vi "Configure Serial Bus (USBP - Trigger).vi"(0 "VISA resource name":refnum<visa-resource-name>, 1 "Control Message Type (0: Good CRC)":i32(ring) items=["Good CRC", "Goto Min", "Accept", "Reject", "Ping", "PS_RDY", "Get Source Cap", "Get Sink Cap", "DR Swap", "PR Swap", " VCONN Swap", "Wait", "Soft Reset", "Get Source Cap Extended ", "Get Status ", "FR Swap", "Get PPS Status ", "Get Country Codes "], 2 "Qualifier Type (0: None)":i32(ring) items=["None", "SOP", "SPR", "SDPR"], 5 "Serial Bus Name (1: Serial Bus 1)":i32(ring)=1 items=["Serial Bus 1"=1, "Serial Bus 2"=2], 7 "Trigger Mode (0: Preamble Start)":i32(ring) items=["Preamble Start", "End Of Packet", "SOP", "SP Rime", "SDP Rime", "SP Debug", "SDP Debug", "Hard Reset", "Cable Reset", "CRC Error", "Preamble Error", "Header Content"], 9 "Header Type (0: Control Message)":i32(ring) items=["Control Message", "Data Message", "Extended Message", " Value"], 11 "error in (no error)":errorcluster, 12 "Data Message Type (0: Source Capabilities)":i32(ring) items=["Source Capabilities", "Request", "BIST", "Sink Capabilities", "Battery Status", "Alert", "Get Country Info", "Vendor Defined"], 13 "Extended Message Type (0: Source Capabilities Extended )":i32(ring) items=["Source Capabilities Extended ", "Status", "Get Battery Cap", "Get Battery Status", "Battery Capabilities", "Get Manufacturer Info", "Manufacturer Info", "Security Request", "Security Response", "Firmware Update Request", "Firmware Update Response", "PPS Status", "Country Information", "Country Codes"], 14 "Header Value (XXXXXXXXXXXXXXXX)":string="XXXXXXXXXXXXXXXX") -> (4 "VISA resource name out":refnum<visa-resource-name>, 15 "error out":errorcluster)   [LabVIEW 2015, in "Agilent 2000 3000 X-Series.lvlib"]
doc: "Configures the trigger settings of USB Pd bus.\n\n<b>Note:</b>\nThis VI is only applicable for 3000T, 3000G, 4000 X-Series."
uses:
  Agilent 2000 3000 X-Series.lvlib
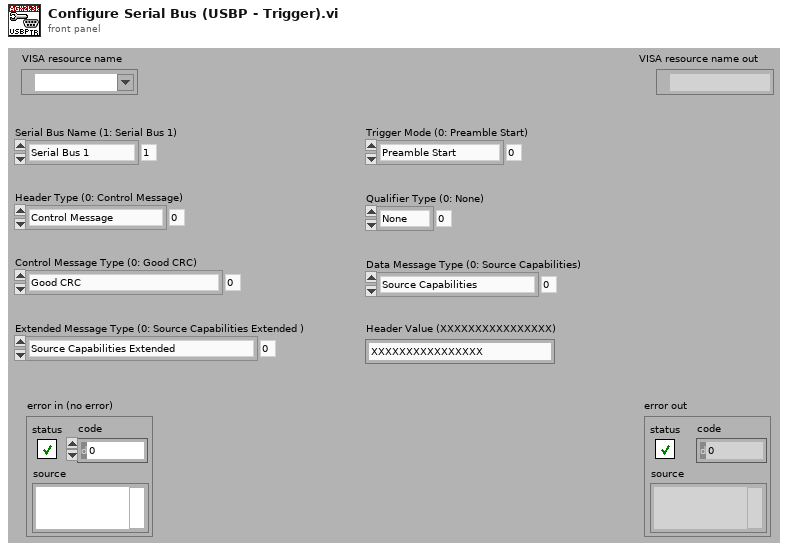
[diagram p1: front panel]
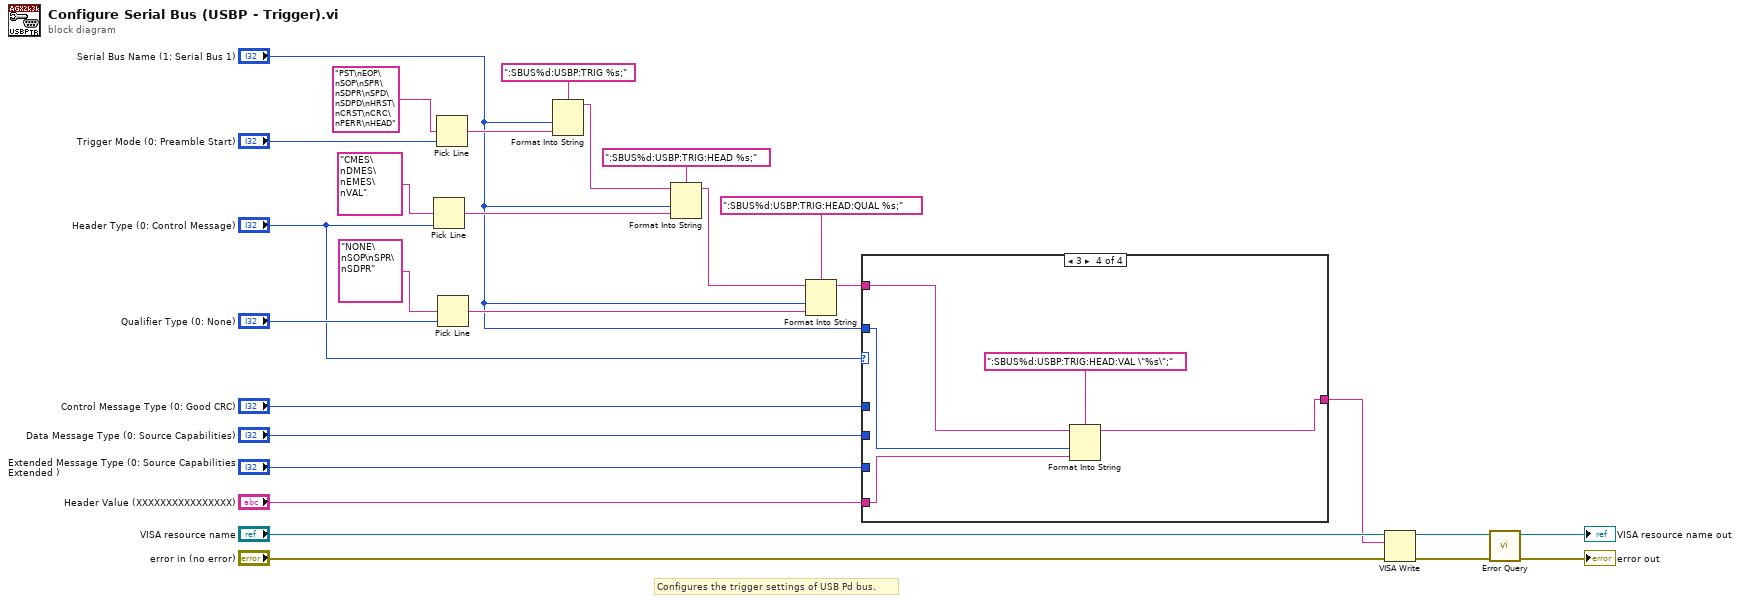
[diagram p0: block diagram]
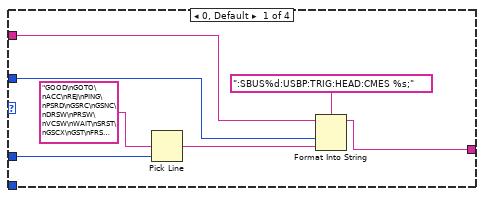
[diagram p2: hidden frame]
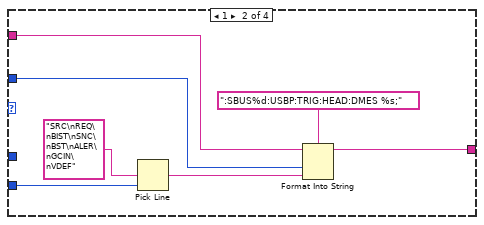
[diagram p3: hidden frame]
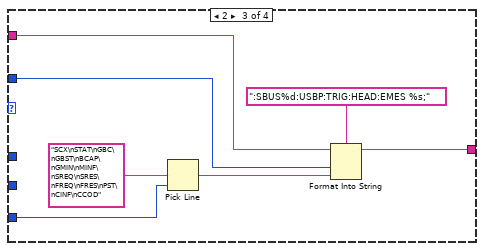
[diagram p4: hidden frame]
diagram:
  # "Configures the trigger settings of USB Pd bus."
  n1 = Pick Line(multi-line string="CMES\nDMES\nEMES\nVAL", line index="Header Type (0: Control Message)") -> (output string=w17:string)  [unwired: 1 in]
  n2 = Pick Line(multi-line string="PST\nEOP\nSOP\nSPR\nSDPR\nSPD\nSDPD\nHRST\nCRST\nCRC\nPERR\nHEAD", line index="Trigger Mode (0: Preamble Start)") -> (output string=w24:string)  [unwired: 1 in]
  n3 = Pick Line(multi-line string="NONE\nSOP\nSPR\nSDPR", line index="Qualifier Type (0: None)") -> (output string=w20:string)  [unwired: 1 in]
  n4 = Format Into String(format string=":SBUS%d:USBP:TRIG %s;", "Serial Bus Name (1: Serial Bus 1)", w24) -> (resulting string=w14:string)  [unwired: 2 in, 1 out]
  n5 = Format Into String(format string=":SBUS%d:USBP:TRIG:HEAD %s;", initial string=w14, "Serial Bus Name (1: Serial Bus 1)", w17) -> (resulting string=w13:string)  [unwired: 1 in, 1 out]
  n6 = Format Into String(format string=":SBUS%d:USBP:TRIG:HEAD:QUAL %s;", initial string=w13, "Serial Bus Name (1: Serial Bus 1)", w20) -> (resulting string=w11:string)  [unwired: 1 in, 1 out]
  n7 = case shown="3" "Header Type (0: Control Message)" {
    tunnel: w11 -> [w31 w36 w44 w50]
    tunnel: "Serial Bus Name (1: Serial Bus 1)" -> [w30 w37 w45 w51]
    tunnel: "Control Message Type (0: Good CRC)" -> [w33 _ _ _]
    tunnel: "Data Message Type (0: Source Capabilities)" -> [_ w38 _ _]
    tunnel: [w29 w35 w42 w49] -> w1
    tunnel: "Extended Message Type (0: Source Capabilities Extended )" -> [_ _ w46 _]
    tunnel: "Header Value (XXXXXXXXXXXXXXXX)" -> [_ _ _ w52]
    frame 0, Default {
      n8 = Pick Line(multi-line string="GOOD\nGOTO\nACC\nREJ\nPING\nPSRD\nGSRC\nGSNC\nDRSW\nPRSW\nVCSW\nWAIT\nSRST\nGSCX\nGST\nFRSW\nGPST\nGCC", line index=w33) -> (output string=w32:string)  [unwired: 1 in]
      n9 = Format Into String(format string=":SBUS%d:USBP:TRIG:HEAD:CMES %s;", initial string=w31, w30, w32) -> (resulting string=w29:string)  [unwired: 1 in, 1 out]
    }
    frame 1 {
      n10 = Pick Line(multi-line string="SRC\nREQ\nBIST\nSNC\nBST\nALER\nGCIN\nVDEF", line index=w38) -> (output string=w41:string)  [unwired: 1 in]
      n11 = Format Into String(format string=":SBUS%d:USBP:TRIG:HEAD:DMES %s;", initial string=w36, w37, w41) -> (resulting string=w35:string)  [unwired: 1 in, 1 out]
    }
    frame 2 {
      n12 = Pick Line(multi-line string="SCX\nSTAT\nGBC\nGBST\nBCAP\nGMIN\nMINF\nSREQ\nSRES\nFREQ\nFRES\nPST\nCINF\nCCOD", line index=w46) -> (output string=w48:string)  [unwired: 1 in]
      n13 = Format Into String(format string=":SBUS%d:USBP:TRIG:HEAD:EMES %s;", initial string=w44, w45, w48) -> (resulting string=w42:string)  [unwired: 1 in, 1 out]
    }
    frame 3 {
      n14 = Format Into String(format string=":SBUS%d:USBP:TRIG:HEAD:VAL \"%s\";", initial string=w50, w51, w52) -> (resulting string=w49:string)  [unwired: 1 in, 1 out]
    }
  }
  n15 = VISA Write(VISA resource name="VISA resource name", write buffer=w1, error in (no error)="error in (no error)") -> (VISA resource name out=w5:refnum<visa-resource-name>, error out=w4:errorcluster)  [unwired: 1 out]
  n16 = call "Error Query.vi"("error in (no error)"=w4, "VISA resource name"=w5) -> ("error out"=→"error out":errorcluster, "VISA resource name out"=→"VISA resource name out":refnum<visa-resource-name>)  [unwired: 6 in, 2 out]
